vi "Pack for gRPC.vi"(8 "error in":errorcluster, 9 "configuration / results":enum16{"Configuration", "Results"}(ring), 10 "data value":variant, 11 "measurement plugin in":refnum<class "FPT_SParam_VST.lvclass">) -> (0 "error out":errorcluster, 2 "any":T1, 3 "measurement plugin out":refnum<class "FPT_SParam_VST.lvclass">)   [LabVIEW 2023, in "FPT_SParam_VST.lvclass"]
uses:
  FPT_SParam_VST.lvclass
  <vilib>/gRPC/LabVIEW gRPC Library/Shared/Any.ctl
  Measurement Configuration.ctl
  Measurement Results.ctl
  2eca732d-dbaa-43bf-a7dd-ede2da65bc1b.vi
  a6012965-5700-4384-8228-972e71b6560c.vi
  <vilib>/gRPC/LabVIEW gRPC Library/Server API/Translate Protobuf Error.vi
  <vilib>/AdvancedString/1D String Array to Delimited String.vi
  <vilib>/gRPC/LabVIEW gRPC Library/Server API/Server/Get Server DLL Path.vi
  FPT_SParam_VST.lvclass/FPT_SParam_VST.ctl
  <vilib>/Plug-In SDKs/Measurements/Measurement Plugin Service/Measurement Plugin Service.lvclass
  <vilib>/gRPC/LabVIEW gRPC Library/grpc-lvsupport-release.lvlib
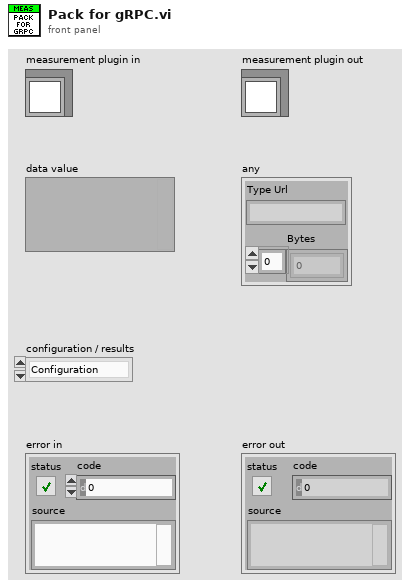
[diagram p1: front panel]
types:
  T1 = typedef "grpc-lvsupport-release.lvlib/Any.ctl" = cluster{"Type Url":string, "Bytes":u8[]}
  T2 = typedef "grpc-lvsupport-release.lvlib/grpcId.ctl" = u64
  T3 = typedef "FPT_SParam_VST.lvclass/Measurement Configuration.ctl" = cluster{"Automation Test":bool, "Power sequencing file path":string, "VST Resource Name":string, "RFSG port":string, "RFmx port":string, "RF Out Switch":string, "Common RFout":string, "Port1 Incident":string, "Port2 Incident":string, "RF In Switch":string, "Common RFin":string, "Port1 Reference":string, "Port1 Test":string, "Port2 Reference":string, "Port2 Test":string, "RFSG attenuation mode":enum32{"<None>", "Constant Attenuation"}, "RFSG external attenuation (dB)":dbl, "Save Calibration File at":string, "Short S1P":string, "Open S1P":string, "Load S1P":string, "Through Adapter S2P":string, "Action":enum32{"Calibrate", "Measure"}, "Power Level (dBm)":dbl, "External Gain (dB)":dbl, "Start Frequency (Hz)":dbl, "Stop Frequency (Hz)":dbl, "Step Size (Hz)":dbl, "Type of Stimulus":enum32{"CW", "Pulsed CW"}, "Pulse Width (s)":dbl, "PRI (s)":dbl, "IF Bandwidth (Hz)":dbl, "Average Mode":enum32{"Per Sweep", "Per Point"}, "Number of Averages":i32, "SnP File Path":string, "Calibration File Path":string, "Power sequencing file validity check":bool}
  T4 = typedef "FPT_SParam_VST.lvclass/Measurement Results.ctl" = cluster{"Status":string, "S-Param Magnitude":dbl[][], "S-Param Phase":dbl[][], "S21 (Mean)":dbl, "S12 (Mean)":dbl}
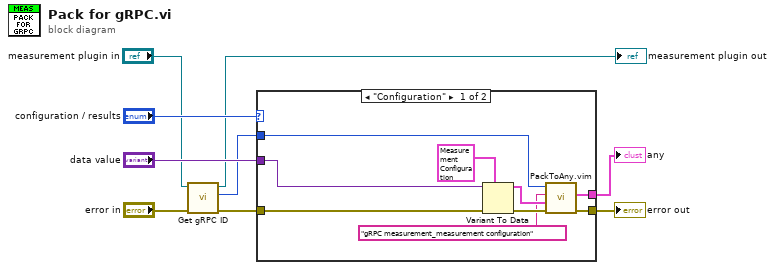
[diagram p0: block diagram]
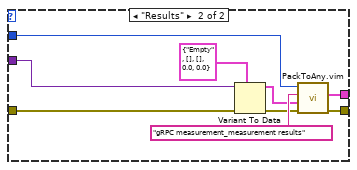
[diagram p2: hidden frame]
diagram:
  n1 = call <vilib>:"Get gRPC ID.vi"("error in"="error in", "measurement plugin service in"="measurement plugin in") -> ("error out"=w4:errorcluster, "gRPC ID"=w1:T2, "measurement plugin service out"=→"measurement plugin out":refnum<class "FPT_SParam_VST.lvclass">)  [unwired: 7 in]
  n2 = case shown="\"Configuration\"" "configuration / results" {
    tunnel: w4 -> [w18 w27]
    tunnel: "data value" -> [w17 w26]
    tunnel: w1 -> [w14 w22]
    tunnel: [w16 w24] -> w8
    tunnel: [w15 w23] -> w7
    frame "Configuration" {
      n3 = Variant To Data(error in=w18, type=T3 {"Automation Test"=FALSE, "Power sequencing file path"="Lorem ipsum dolor sit", "VST Resource Name"="5842_0", "RFSG port"="", "RFmx port"="", "RF Out Switch"="", "Common RFout"="", "Port1 Incident"="", "Port2 Incident"="", "RF In Switch"="", "Common RFin"="", "Port1 Reference"="", "Port1 Test"="", "Port2 Reference"="", "Port2 Test"="", "RFSG attenuation mode"=enum."Constant Attenuation", "RFSG external attenuation (dB)"=1.0, "Save Calibration File at"="", "Short S1P"="", "Open S1P"="", "Load S1P"="", "Through Adapter S2P"="", "Action"=enum."Measure", "Power Level (dBm)"=1.0, "External Gain (dB)"=2e-05, "Start Frequency (Hz)"=4000000000.0, "Stop Frequency (Hz)"=26000000000.0, "Step Size (Hz)"=0.0, "Type of Stimulus"=enum."Pulsed CW", "Pulse Width (s)"=0.0, "PRI (s)"=0.0, "IF Bandwidth (Hz)"=1.0, "Average Mode"=enum."Per Sweep", "Number of Averages"=0, "SnP File Path"="", "Calibration File Path"="", "Power sequencing file validity check"=TRUE} ("measurement configuration"), Variant=w17) -> (data=w13:T3, error out=w12:errorcluster)
      n4 = call "PackToAny.vim"("error in"=w12, "Data To Pack"=w13, "Message Type"="gRPC measurement_measurement configuration", "gRPCid in"=w14) -> ("error out"=w16:errorcluster, "Any"=w15:T1)  [unwired: 5 in, 1 out]
    }
    frame "Results" {
      n5 = Variant To Data(error in=w27, type=T4 {"Status"="Empty", "S-Param Magnitude"=[], "S-Param Phase"=[], "S21 (Mean)"=0.0, "S12 (Mean)"=0.0} ("Measurement Results"), Variant=w26) -> (data=w20:T4, error out=w19:errorcluster)
      n6 = call "PackToAny.vim"("error in"=w19, "Data To Pack"=w20, "Message Type"="gRPC measurement_measurement results", "gRPCid in"=w22) -> ("error out"=w24:errorcluster, "Any"=w23:T1)  [unwired: 5 in, 1 out]
    }
  }
  "error out" <- w8
  "any" <- w7
